vi "TENMA 72-2930 general control.vi"(6 "Value to set":sgl, 7 "Command":T1="*IDN?", 8 "Port":refnum<visa-resource-name>) -> (0 "Output enabled":bool, 1 "error out":errorcluster, 2 "CV mode":bool, 3 "Returned string":string, 5 "Returned value":sgl=nan format="%_4g")   [LabVIEW 2018]
uses:
  ctls/TENMA 72-2xxx commands.ctl
  <vilib>/Instr/_visa.llb/VISA Open Access Mode.ctl
panel:
  # "PN 19/04/18"
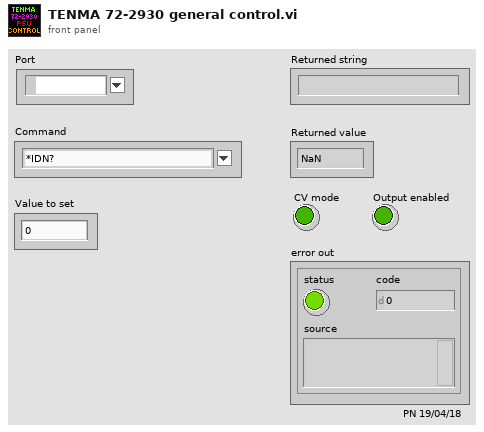
[diagram p1: front panel]
types:
  T1 = typedef "TENMA 72-2xxx commands.ctl" = string
  T2 = typedef "VISA Open Access Mode.ctl" = u32
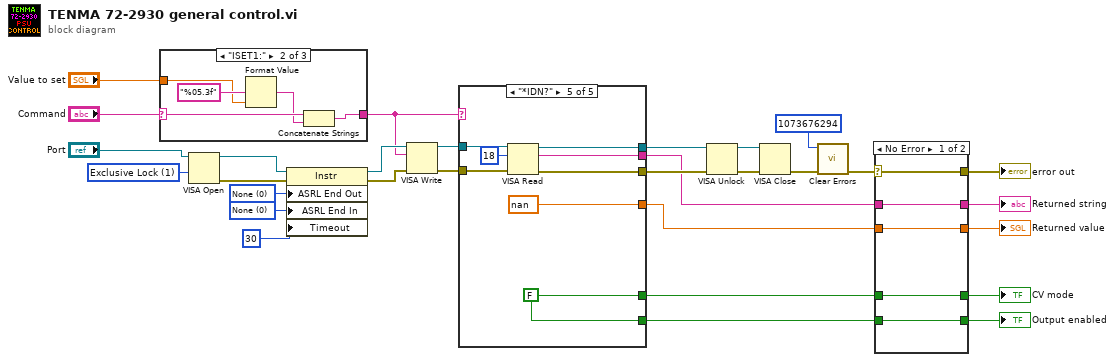
[diagram p0: block diagram]
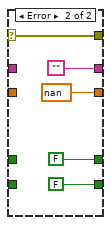
[diagram p2: hidden frame]
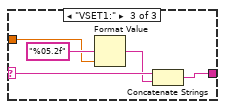
[diagram p4: hidden frame]
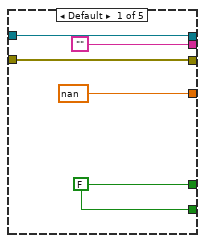
[diagram p5: hidden frame]
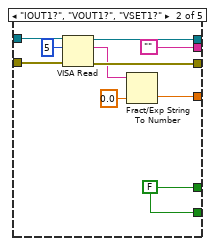
[diagram p6: hidden frame]
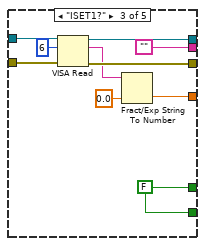
[diagram p7: hidden frame]
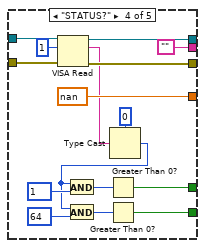
[diagram p8: hidden frame]
diagram:
  w19 = u16 0 items=["None", "Last Bit", "TermChar"] ("Serial Settings:End Mode for Reads")
  w20 = u16 0 items=["None", "Last Bit", "TermChar", "Break"] ("Serial Settings:End Mode for Writes")
  w30 = T2 1 items=["VISA Defaults"=0, "Exclusive Lock"=1, "Load Configured Settings"=4] ("Access Mode")
  n1 = case shown="\"ISET1:\"" "Command" {
    selector: "Command" -> [w31 w36 w41]
    tunnel: [w31 w35 w40] -> w13
    tunnel: "Value to set" -> [_ w33 w38]
    frame Default {
    }
    frame "ISET1:" {
      n2 = Format Value(format string="%05.3f", value (0)=w33) -> (output string=w32:string)  [unwired: 1 in]
      n3 = Concatenate Strings(w36, w32) -> (w35:string)
    }
    frame "VSET1:" {
      n4 = Format Value(format string="%05.2f", value (0)=w38) -> (output string=w37:string)  [unwired: 1 in]
      n5 = Concatenate Strings(w41, w37) -> (w40:string)
    }
  }
  n6 = VISA Open(access mode=w30, VISA resource name="Port") -> (VISA resource name=w24:refnum<visa-resource-name>, error out=w22:errorcluster)  [unwired: 3 in]
  n7 = property class="Instr"(reference=w24, error in=w22, "ASRL End Out"=w20, "ASRL End In"=w19, "Timeout"=u32 30 ("General Settings:Timeout Value")) -> (reference out=w23:refnum<visa-resource-name>, error out=w21:errorcluster)
  n8 = VISA Write(VISA resource name=w23, write buffer=w13, error in (no error)=w21) -> (VISA resource name out=w16:refnum<visa-resource-name>, error out=w15:errorcluster)  [unwired: 1 out]
  n9 = case shown="\"*IDN?\"" w13 {
    tunnel: [w45 w56 w66 w82 w90] -> w26
    tunnel: [w46 w55 w65 w81 w89] -> w25
    tunnel: ["" "" "" "" w88] -> w9
    tunnel: w16 -> [w46 w54 w64 w80 w87]
    tunnel: w15 -> [w45 w53 w63 w79 w86]
    tunnel: [sgl nan w49 w59 sgl nan sgl nan] -> w8
    tunnel: [w42 w47 w57 w71 w83] -> w7
    tunnel: [w42 w47 w57 w67 w83] -> w6
    frame Default {
      w42 = FALSE
    }
    frame "IOUT1?", "VOUT1?", "VSET1?" {
      w47 = FALSE
      n10 = VISA Read(VISA resource name=w54, byte count=u32 5, error in (no error)=w53) -> (VISA resource name out=w55:refnum<visa-resource-name>, read buffer=w51:string, error out=w56:errorcluster)  [unwired: 1 out]
      n11 = Fract/Exp String To Number(string=w51, default (0 dbl)=sgl 0.0 ("default (0 DBL)")) -> (number=w49:sgl)  [unwired: 2 in, 1 out]
    }
    frame "ISET1?" {
      w57 = FALSE
      n12 = VISA Read(VISA resource name=w64, byte count=u32 6, error in (no error)=w63) -> (VISA resource name out=w65:refnum<visa-resource-name>, read buffer=w61:string, error out=w66:errorcluster)  [unwired: 1 out]
      n13 = Fract/Exp String To Number(string=w61, default (0 dbl)=sgl 0.0 ("default (0 DBL)")) -> (number=w59:sgl)  [unwired: 2 in, 1 out]
    }
    frame "STATUS?" {
      n14 = VISA Read(VISA resource name=w80, byte count=u32 1, error in (no error)=w79) -> (VISA resource name out=w81:refnum<visa-resource-name>, read buffer=w76:string, error out=w82:errorcluster)  [unwired: 1 out]
      n15 = Type Cast(type=u8 0, x=w76) -> (*(type *) &x=w70:u8)
      n16 = And(x=w70, y=u8 1) -> (x .and. y?=w72:u8)
      n17 = And(x=w70, y=u8 64) -> (x .and. y?=w68:u8)
      n18 = Greater Than 0?(x=w72) -> (x > 0?=w71:bool)
      n19 = Greater Than 0?(x=w68) -> (x > 0?=w67:bool)
    }
    frame "*IDN?" {
      w83 = FALSE
      n20 = VISA Read(VISA resource name=w87, byte count=u32 18, error in (no error)=w86) -> (VISA resource name out=w89:refnum<visa-resource-name>, read buffer=w88:string, error out=w90:errorcluster)  [unwired: 1 out]
    }
  }
  n21 = VISA Unlock(8:w26, 11:w25) -> (0:w29:errorcluster, 3:w28:refnum<visa-resource-name>)
  n22 = VISA Close(VISA resource name=w28, error in (no error)=w29) -> (error out=w27:errorcluster)
  n23 = call <vilib>:"Clear Errors.vi"("error in (no error)"=w27, "specific error code to clear (0: all)"=1073676294) -> ("error out"=w11:errorcluster)  [unwired: 4 in, 1 out]
  n24 = case shown="No Error" w11 {
    selector: w11 -> [w95 w100]
    tunnel: [w95 w100] -> w10
    tunnel: w9 -> [w94 _]
    tunnel: w8 -> [w93 _]
    tunnel: w7 -> [w92 _]
    tunnel: w6 -> [w91 _]
    tunnel: [w94 ""] -> w5
    tunnel: [w93 sgl nan] -> w4
    tunnel: [w92 FALSE] -> w3
    tunnel: [w91 FALSE] -> w2
    frame No Error {
    }
    frame Error {
    }
  }
  "error out" <- w10
  "Returned string" <- w5
  "Returned value" <- w4
  "CV mode" <- w3
  "Output enabled" <- w2
